vi "12_Cave_Create.vi"(8 "Error In":errorcluster, 10 "Name":string, 11 "reference in":refnum<class "12_Cave.lvclass">) -> (0 "Error Out":errorcluster, 3 "reference out":refnum<class "12_Cave.lvclass">)   [LabVIEW 2020, in "12_Cave.lvclass"]
uses:
  12_Cave.lvclass
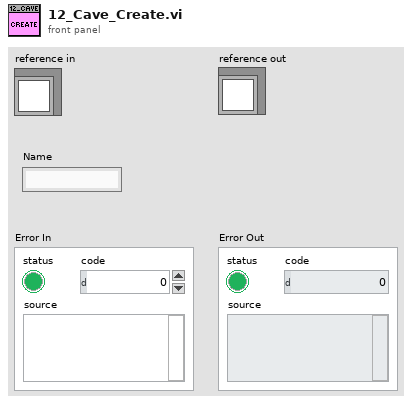
[diagram p1: front panel]
types:
  T1 = typedef "12_Cave.lvclass/ObjectAttributes.ctl" = cluster{"Neighbours":refnum<class "12_Cave.lvclass">[], "Is Big":bool, "Name":string}
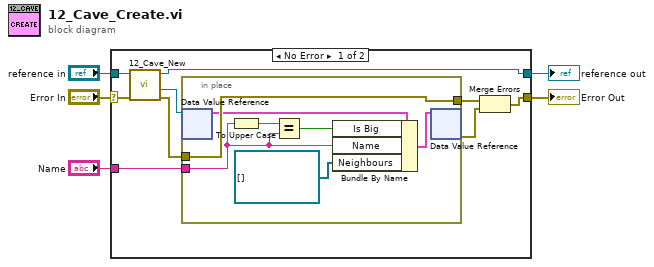
[diagram p0: block diagram]
diagram:
  n1 = case shown="No Error" "Error In" {
    selector: "Error In" -> [w13 w23]
    tunnel: [w7 w23] -> w4
    tunnel: "reference in" -> [w14 w22]
    tunnel: [w12 w22] -> w2
    tunnel: "Name" -> [w6 _]
    frame No Error {
      n2 = call "12_Cave_New.vi"("error in (no error)"=w13, "reference in"=w14) -> ("error out"=w9:errorcluster, "DVRRefOut"=w10:refnum<data-value>, "reference out"=w12:refnum<class "12_Cave.lvclass">)  [unwired: 6 in, 1 out]
      n3 = in-place {
        in-place-border: w9 -> [w21]
        in-place-border: [w21] -> w8
        in-place-border: w6 -> [w17]
        n4 = in-place-dvr #1(w10) -> (w20:T1)  [unwired: 1 out]
        n5 = To Upper Case(1:w17) -> (0:w18:string)
        n6 = Equal?(x=w18, y=w17) -> (x = y?=w16:bool)
        n7 = Bundle By Name(cluster=w20, "Is Big"=w16, "Name"=w17, "Neighbours"=refnum<class "12_Cave.lvclass">[] []) -> (w19:T1)
        n8 = in-place-dvr #1(w19) -> (w11:errorcluster)  [unwired: 1 out]
      }
      n9 = Merge Errors(w8, w11) -> (w7:errorcluster)
    }
    frame Error {
      # "VI-TechBaseTemplate_Simple_4x4x4"
    }
  }
  "Error Out" <- w4
  "reference out" <- w2
